vi "Equalise_aspect_ratio.vi"(3 "error in (no error)":errorcluster, 4 "minmax":dbl[](array[numeric]), 5 "ref in":refnum<vi>) -> (0 "error out":errorcluster, 1 "ratio":dbl, 2 "ref out":refnum<vi>)   [LabVIEW 2010]
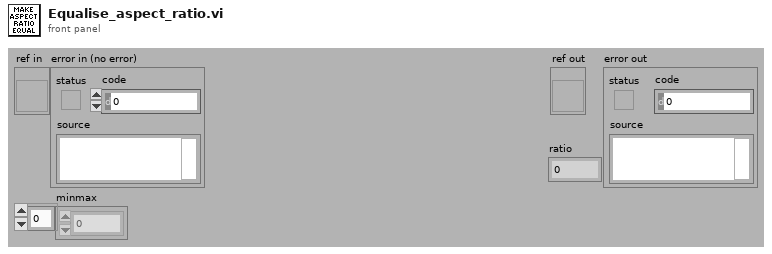
[diagram p1: front panel]
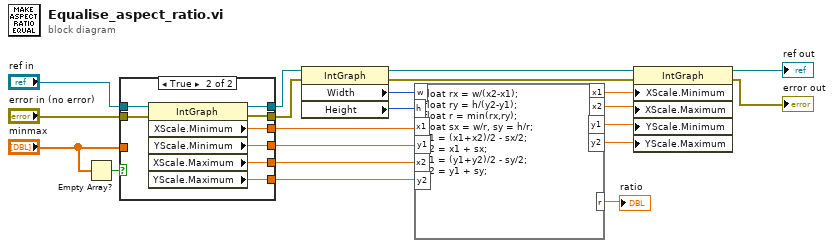
[diagram p0: block diagram]
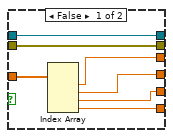
[diagram p2: hidden frame]
diagram:
  n1 = Empty Array?(array="minmax") -> (empty?=w10:bool)
  n2 = case shown="True" w10 {
    tunnel: "minmax" -> [w28 _]
    tunnel: "ref in" -> [w22 w36]
    tunnel: [w22 w35] -> w7
    tunnel: [w23 w34] -> w8
    tunnel: [w27 w33] -> w5
    tunnel: [w26 w32] -> w4
    tunnel: [w25 w31] -> w3
    tunnel: [w24 w30] -> w2
    tunnel: "error in (no error)" -> [w23 w29]
    frame False {
      n3 = Index Array(array=w28) -> (element #1=w27:dbl, element #2=w26:dbl, element #3=w25:dbl, element #4=w24:dbl)  [unwired: 4 in]
    }
    frame True {
      n4 = property class="IntGraph"(reference=w36, error in=w29) -> (reference out=w35:refnum<vi>, error out=w34:errorcluster, "XScale.Minimum"=w33:dbl, "YScale.Minimum"=w32:dbl, "XScale.Maximum"=w31:dbl, "YScale.Maximum"=w30:dbl)
    }
  }
  n5 = property class="IntGraph"(reference=w7, error in=w8) -> (reference out=w15:refnum<vi>, error out=w1:errorcluster, "Width"=w21:u32, "Height"=w20:u32)
  n6 = formula code="float rx = w/(x2-x1);\nfloat ry = h/(y2-y1);\nfloat r = min(rx,ry);\nfloat sx = w/r, sy = h/r;\nx1 = (x1+x2)/2 - sx/2;\nx2 = x1 + sx;\ny1 = (y1+y2)/2 - sy/2;\ny2 = y1 + sy;"("w"=w21, "h"=w20, "x1"=w5, "y1"=w4, "x2"=w3, "y2"=w2) -> ("x1"=w19:dbl, "x2"=w18:dbl, "y1"=w16:dbl, "y2"=w17:dbl, "r"=→"ratio":dbl)
  n7 = property class="IntGraph"(reference=w15, error in=w1, "XScale.Minimum"=w19, "XScale.Maximum"=w18, "YScale.Minimum"=w16, "YScale.Maximum"=w17) -> (reference out=→"ref out":refnum<vi>, error out=→"error out":errorcluster)
